vi "PenaltyDefenseRole.vi"(8 "error in (no error)":errorcluster, 10 "IndexInVector":dbl, 11 "PenaltyDefenseRole in":refnum<class "PenaltyDefenseRole.lvclass">) -> (0 "error out":errorcluster, 2 "Robot out":refnum<class "Robot.lvclass">, 3 "PenaltyDefenseRole out":refnum<class "PenaltyDefenseRole.lvclass">)   [LabVIEW 2023, in "PenaltyDefenseRole.lvclass"]
uses:
  PenaltyDefenseRole.lvclass
  Robot_class/Robot.lvclass
  Game_class/Game.lvclass
  Role_class/Role.lvclass/Role.ctl
  Tacticbook_class/Tacticbook.lvclass/Tacticbook.ctl
  Tacticbook_class/Read PenaltyDefenseTactic.vi
  PenaltyDefenseTactic_class/Read States.vi
  Tacticbook_class/Write PenaltyDefenseTactic.vi
  Role_class/Read Tacticbook.vi
  Role_class/Read tactic_index.vi
  Role_class/Write Tacticbook.vi
  Role_class/Write tactic_index.vi
  Role_class/Read RobotRef.vi
  Tacticbook_class/Tacticbook.lvclass
  PenaltyDefenseTactic_class/PenaltyDefenseTactic.lvclass
panel:
  out "Game out":refnum<class "Game.lvclass">
  in  "Game in":refnum<class "Game.lvclass">
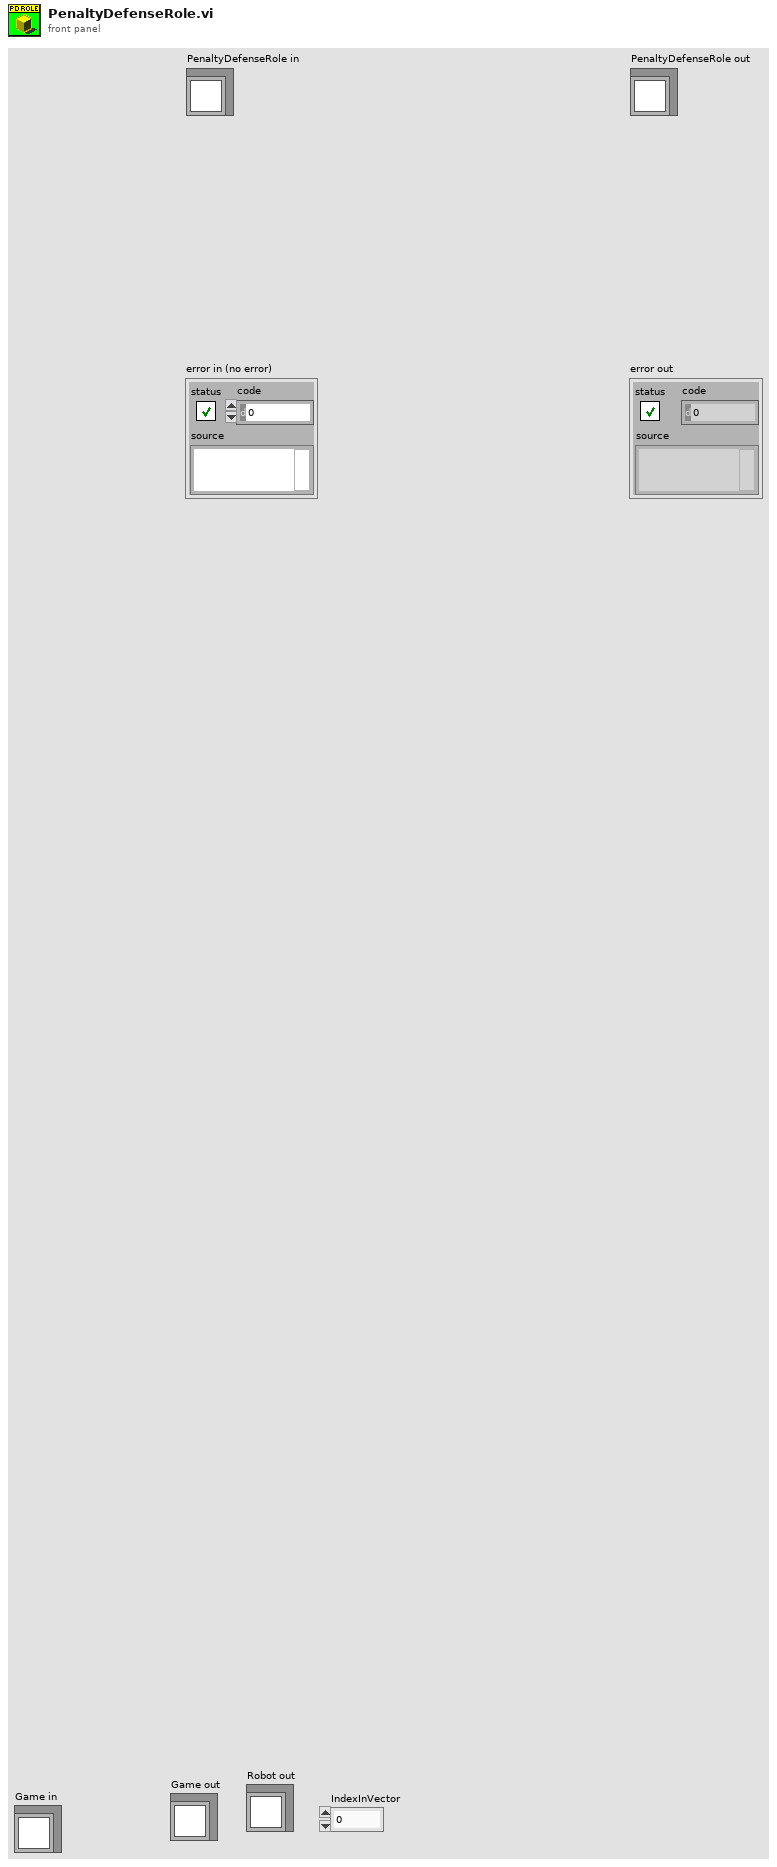
[diagram p1: front panel]
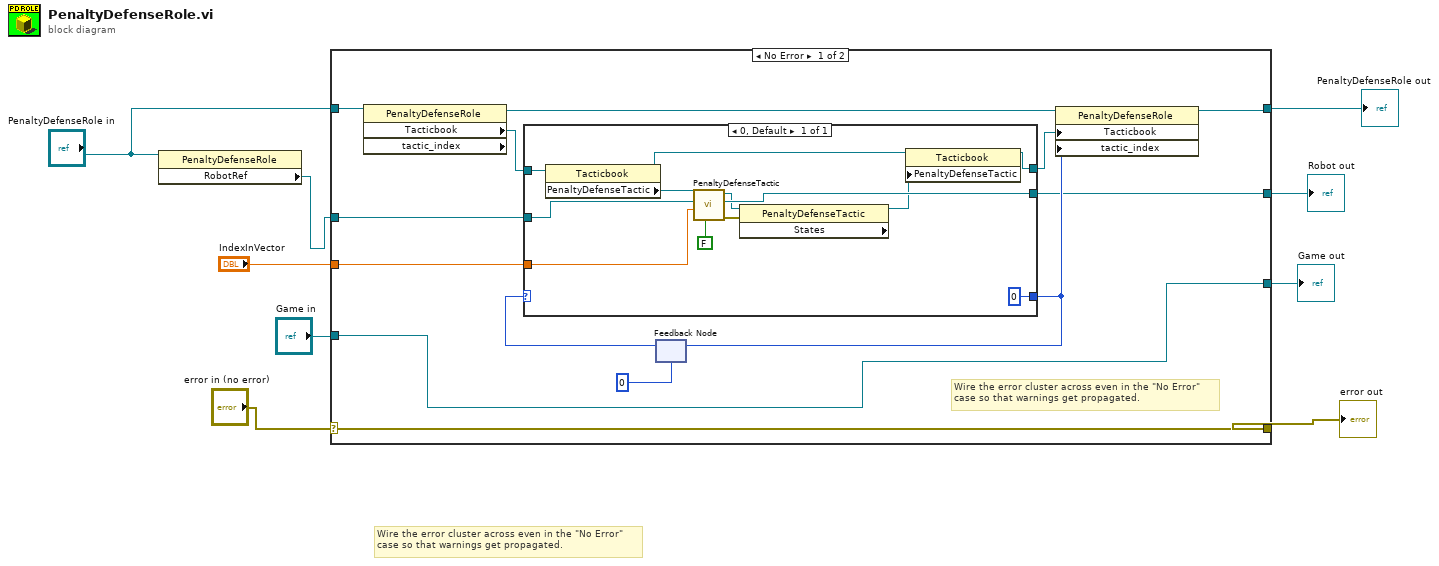
[diagram p0: block diagram]
diagram:
  # "Wire the error cluster across even in the \"No Error\"\ncase so that warnings get propagated."
  n1 = property class="PenaltyDefenseRole"(reference="PenaltyDefenseRole in") -> ("RobotRef"=w6:refnum<class "Robot.lvclass">)  [unwired: 1 in, 2 out]
  n2 = case shown="No Error" "error in (no error)" {
    selector: "error in (no error)" -> [w22 w38]
    tunnel: [w22 w38] -> w3
    tunnel: [w20 w37] -> w4
    tunnel: "PenaltyDefenseRole in" -> [w21 w37]
    tunnel: w6 -> [w14 w36]
    tunnel: [w13 w36] -> w8
    tunnel: [w11 w35] -> w7
    tunnel: "Game in" -> [w11 w35]
    tunnel: "IndexInVector" -> [w10 _]
    frame No Error {
      # "Wire the error cluster across even in the \"No Error\"\ncase so that warnings get propagated."
      n3 = property class="PenaltyDefenseRole" props=["Tacticbook", "tactic_index"](reference=w21) -> (reference out=w19:refnum<class "PenaltyDefenseRole.lvclass">, "Tacticbook"=w16:refnum<class "Tacticbook.lvclass">)  [unwired: 1 in, 2 out]
      n4 = feedback #1(0) -> (w17:i32)
      n5 = case shown="0, Default" w17 {
        tunnel: [0] -> w15
        tunnel: w16 -> [w34]
        tunnel: w14 -> [w27]
        tunnel: [w33] -> w13
        tunnel: [w29] -> w12
        tunnel: w10 -> [w23]
        frame 0, Default {
          n6 = property class="Tacticbook"(reference=w34) -> (reference out=w31:refnum<class "Tacticbook.lvclass">, "PenaltyDefenseTactic"=w28:refnum<class "PenaltyDefenseTactic.lvclass">)  [unwired: 1 in, 1 out]
          n7 = call-dynamic "PenaltyDefenseTactic.vi"("PenaltyOurKick?"=FALSE, "IndexInVector"=w23, "Robot"=w27, "PenaltyDefenseTactic in"=w28) -> ("error out"=w32:errorcluster, "Robot out"=w33:refnum<class "Robot.lvclass">, "PenaltyDefenseTactic out"=w26:refnum<class "PenaltyDefenseTactic.lvclass">)  [unwired: 5 in]
          n8 = property class="PenaltyDefenseTactic" props=["States"](reference=w26, error in=w32) -> (reference out=w30:refnum<class "PenaltyDefenseTactic.lvclass">)  [unwired: 2 out]
          n9 = property class="Tacticbook"(reference=w31, "PenaltyDefenseTactic"=w30) -> (reference out=w29:refnum<class "Tacticbook.lvclass">)  [unwired: 1 in, 1 out]
        }
      }
      n10 = feedback-in #1(w15) -> ()
      n11 = property class="PenaltyDefenseRole"(reference=w19, "Tacticbook"=w12, "tactic_index"=w15) -> (reference out=w20:refnum<class "PenaltyDefenseRole.lvclass">)  [unwired: 1 in, 1 out]
    }
    frame Error {
    }
  }
  "error out" <- w3
  "PenaltyDefenseRole out" <- w4
  "Robot out" <- w8
  "Game out" <- w7
